vi "Send CCD Initialization.vi"(8 "error in (no error)":errorcluster, 11 "RxTx in":refnum<class "RxTx.lvclass">) -> (0 "error out":errorcluster, 3 "RxTx out":refnum<class "RxTx.lvclass">)   [LabVIEW 2018, in "RxTx.lvclass"]
uses:
  RxTx.lvclass
  RxTx.lvclass/RxTx.ctl
  Interface/Interface.lvclass/Interface.ctl
  Interface/Interface.lvclass
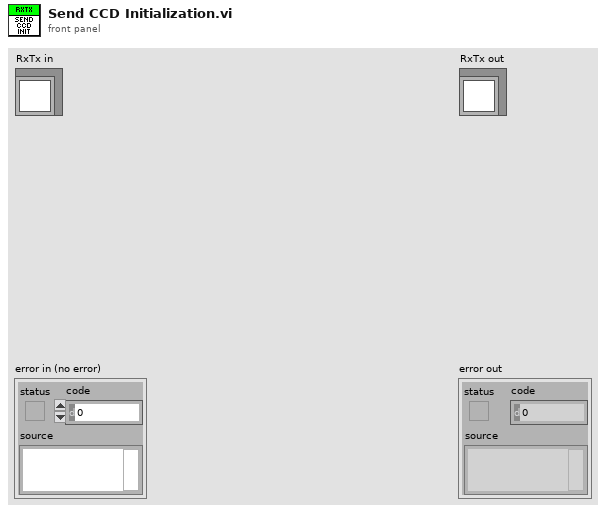
[diagram p1: front panel]
types:
  T1 = cluster{"Initialization":bool, "Serial Number":u16}
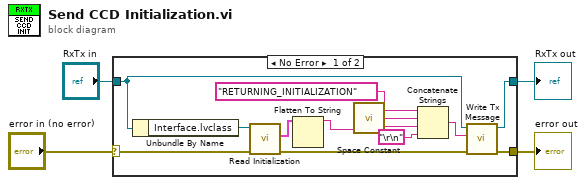
[diagram p0: block diagram]
diagram:
  n1 = case shown="No Error" "error in (no error)" {
    selector: "error in (no error)" -> [w15 w18]
    tunnel: [w9 w18] -> w2
    tunnel: [w10 w17] -> w1
    tunnel: "RxTx in" -> [w11 w17]
    frame No Error {
      n2 = Unbundle By Name(w11) -> ("Interface.lvclass"=w16:refnum<class "Interface.lvclass">)
      n3 = call "Read Initialization.vi"("error in (no error)"=w15, "Interface in"=w16) -> ("error out"=w13:errorcluster, "Initialization"=w6:T1)  [unwired: 7 in, 1 out]
      n4 = Flatten To String(anything=w6) -> (data string=w14:string)  [unwired: 3 in, 2 out]
      n5 = call <vilib>:"Space Constant.vi"() -> ("String"=w7:string)
      n6 = Concatenate Strings("RETURNING_INITIALIZATION", w7, w14, "\r\n") -> (w12:string)
      n7 = call "Write Tx Message.vi"("error in (no error)"=w13, "Tx Message"=w12, "RxTx in"=w11) -> ("error out"=w9:errorcluster, "RxTx out"=w10:refnum<class "RxTx.lvclass">)  [unwired: 7 in]
    }
    frame Error {
    }
  }
  "error out" <- w2
  "RxTx out" <- w1
